vi "GetFileVersion.vi"(10 "path":path) -> (3 "Full version":string)   [LabVIEW 2017]
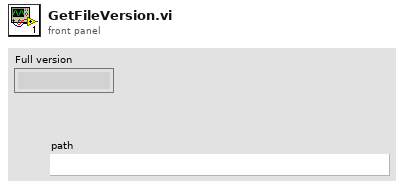
[diagram p1: front panel]
types:
  T1 = enum32{"invalid app kind", "Development System", "Run Time System", "Student Edition", "Embedded LabVIEW", "Evaluation", "Custom"}
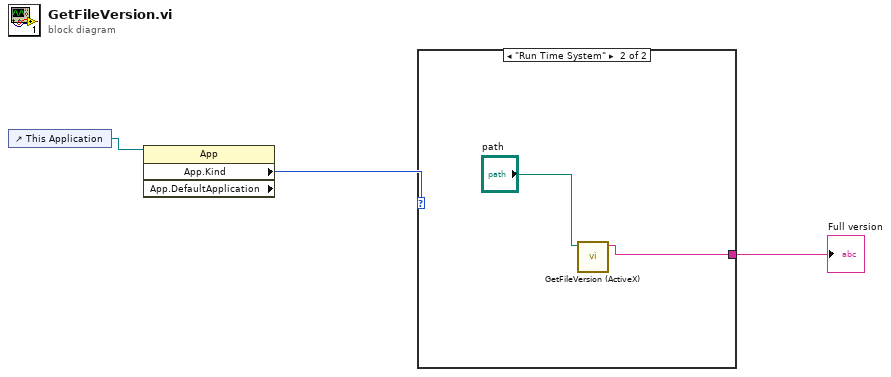
[diagram p0: block diagram]
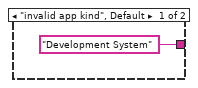
[diagram p2: hidden frame]
diagram:
  n1 = control-ref of="This Application"() -> (w1:refnum<vi>)
  n2 = property class="App" props=["App.Kind", "App.DefaultApplication"](reference=w1) -> ("App.Kind"=w3:T1)  [unwired: 1 in, 3 out]
  n3 = case shown="\"Run Time System\"" w3 {
    tunnel: ["Development System" ("Full version") w5] -> w2
    frame "invalid app kind", Default {
    }
    frame "Run Time System" {
      n4 = call "GetFileVersion (ActiveX).vi"("Filespec"="path") -> ("Full version"=w5:string)  [unwired: 7 in, 3 out]
    }
  }
  "Full version" <- w2
